vi "Camera controle_PID_CL.vi"() -> ()   [LabVIEW 2026]
uses:
  <vilib>/Serenial/G Industrial Camera/g_industrial_cam/Device Enumeration.ctl
  <vilib>/Serenial/G Industrial Camera/g_industrial_cam/Buffer/Image Size.ctl
  C:/Users/laserfab/Desktop/Cam-PID-LV2026/Thorlabs.MotionControl.Controls.dll
  Thorlabs.MotionControl.Controls.dll
  C:/Users/laserfab/Desktop/Cam-PID-LV2026/Thorlabs.MotionControl.TCube.PiezoCLI.dll
  Thorlabs.MotionControl.TCube.PiezoCLI.dll
  Etat-Data.ctl
  Etat.ctl
  Data-Processing.ctl
  <vilib>/Serenial/G Industrial Camera/g_industrial_cam/Buffer/Buffer.lvclass
  <vilib>/Serenial/G Industrial Camera/g_industrial_cam/Camera/Camera.lvclass
  <vilib>/picture/picture.llb/imagedata.ctl
  Data PID.ctl
  Etat_PID.ctl
  Data Process PID.ctl
  <vilib>/Serenial/G Industrial Camera/g_industrial_cam/Camera/Camera.lvclass/Camera.ctl
  <vilib>/Serenial/G Industrial Camera/g_industrial_cam/Buffer/Buffer.lvclass/Buffer.ctl
  Set CX_CY.ctl
  <vilib>/Serenial/G Industrial Camera/g_industrial_cam/Buffer/Read as Pixmap Mono8.vi
  215a0117-6493-43a3-86db-3e9176a583aa.vi
  <vilib>/Serenial/G Industrial Camera/g_industrial_cam/Camera/GetSetGain.vi
  <vilib>/Serenial/G Industrial Camera/g_industrial_cam/Camera/GetSetExposureTime.vi
  <vilib>/Serenial/G Industrial Camera/g_industrial_cam/Buffer/ReadAsPixmapCore.vi
  <vilib>/Serenial/G Industrial Camera/g_industrial_cam/Camera/Check Not Disconnected.vi
  <vilib>/Utility/error.llb/Error Cluster From Error Code.vi
  <vilib>/Serenial/G Industrial Camera/g_industrial_cam/g_industrial_cam.lvlib
panel:
  out "Refnum de .NET en sortie":refnum<k24>
  out "Acquired Frames/s":dbl=20.37037037037037
  in  "Reset PID 2":bool
  in  "dt (s) PID Axe Y":dbl=0.1 format="%#_13g"
  out "Set CY":dbl=230.26622030324862
  out "CY-offset":dbl=-0.06108959017157645
  in  "Switch Axe Y":bool=TRUE
  in  "PID gains Axe Y":T1={"proportional gain (Kc)"=1.2, "integral time (Ti, min)"=0.01, "derivative time (Td, min)"=0.0}
  in  "Switch Axe X":bool=TRUE
  in  "dt (s) PID Axe X":dbl=0.1 format="%#_13g"
  in  "Activer T-CUbe":bool
  in  "Reset PID":bool
  in  "Activer PID":bool
  out "Set CX":dbl=266.3771356699901
  in  "PID gains Axe X":T1={"proportional gain (Kc)"=0.8, "integral time (Ti, min)"=0.01, "derivative time (Td, min)"=0.0}
  out "CX-offset":dbl=-0.033756492270526905
  in  "Commande onglets":T2(tab)=enum."T-Cube"
  out "Image Caméra":i16[][](graph)
  out "Image ROI":i16[][](graph)
  out "moy Y":dbl=0.005019843768275564 format="%0.4f"
  out "centroid X":dbl(graph)=0.040067485170311556
  out "Centroid Y":dbl(graph)=-0.06325731870961704
  out "sigma X":dbl=0.1236529790065538 caption="écart-type X" format="%0.4f"
  out "moy X":dbl=0.031771673220847445 format="%0.4f"
  out "sigma Y":dbl=0.10913064949168795 caption="écart-type Y" format="%0.4f"
  in  "Pixel size(um)":dbl=5.6
  in  "foc lentille(m)":dbl=1.0
  in  "Switch Pix/urad":bool
  in  "nbre pts sigma":i32=2000
  in  "TCube Axe Y":refnum<k24>(container)
  in  "TCube Axe X":refnum<k24>(container)
  in  "SerialNumber Axe X":string="81843305"
  in  "SerialNumber Axe Y":string="81844014"
  out "Tension Sortie PID Axe Y":dbl(graph)=26.251050201925793
  out "Tension Sortie PID Axe X":dbl(graph)
  in  "Bruit de fond":bool
  out "Sensor Size":T3={"Width"=659, "Height"=494}
  in  "Set Centroid":bool
  in  "Shutter (us)":dbl(knob)=1000.0 scale=22.0..10000000.0
  in  "Save Image":bool
  in  "Gain Caméra":i32(knob)=2 scale=0.0..1023.0
  in  "Start /Stop Acquisition":bool
  out "Etat":string="Programme Arrêté"
  out "Devices":T4[](array[typedef])=[{"ID"="Basler-acA640-121gm-40025274", "Protocol"="GigEVision", "Vendor"="Basler", "Model"="acA640-121gm", "Serial"="40025274", "Address"="192.168.3.4"}, {"ID"="Basler-acA640-121gm-40135516", "Protocol"="GigEVision", "Vendor"="Basler", "Model"="acA640-121gm", "Serial"="40135516", "Address"="192.168.3.3"}]
  in  "stop":bool
  out "error out":errorcluster
  # "Commande PID"
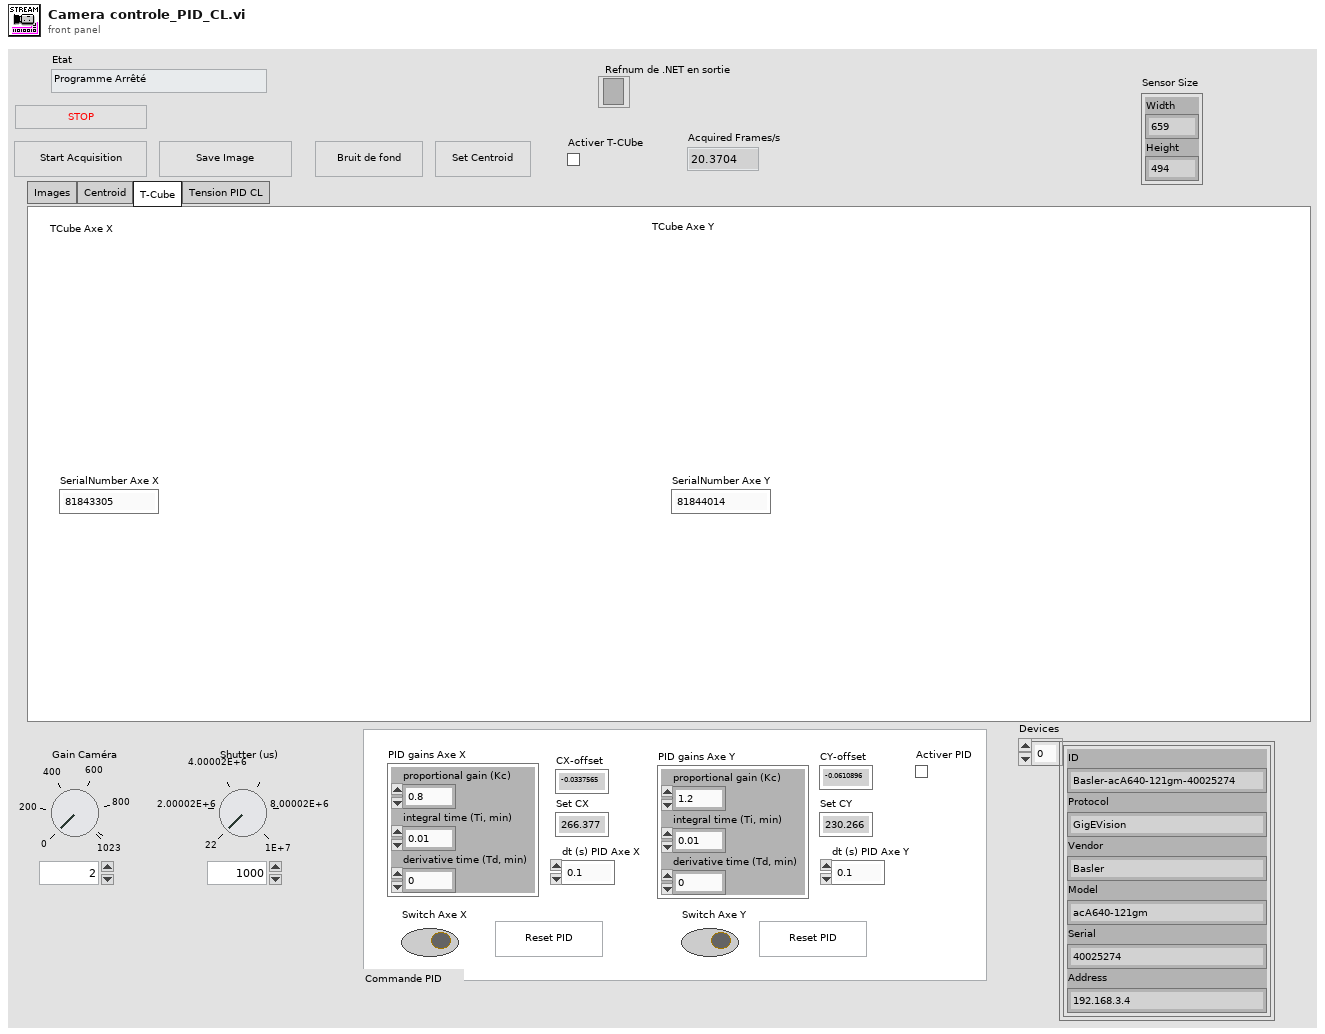
[diagram p1: front panel]
types:
  T1 = cluster{"proportional gain (Kc)":dbl, "integral time (Ti, min)":dbl, "derivative time (Td, min)":dbl}
  T2 = enum32{"Images", "Centroid", "T-Cube", "Tension PID CL"}
  T3 = typedef "g_industrial_cam.lvlib/Buffer.lvclass/Image Size.ctl" = cluster{"Width":u16, "Height":u16}
  T4 = typedef "g_industrial_cam.lvlib/Device Enumeration.ctl" = cluster{"ID":string, "Protocol":string, "Vendor":string, "Model":string, "Serial":string, "Address":string}
  T5 = typedef "Data Process PID.ctl" = cluster{"Pos Init CX":dbl, "Pos Init CY":dbl}
  T6 = typedef "Data PID.ctl" = cluster{"Etat PID":T7, "Data PID":variant}
  T7 = typedef "Etat_PID.ctl" = enum16{"PID", "Stop", "Reset PID", "Set Centroid", "Set T-Cube"}
  T8 = typedef "Data-Processing.ctl" = cluster{"Acqu?":bool, "Image Caméra":picture, "Image Data":T9, "Image brut":i16[][], "BKG":i16[][], "Image -BKG":i16[][], "Offset Centroid X":dbl, "Offset Centroid Y":dbl, "Centroid X-offset":dbl, "Centroid Y-offset":dbl, "Refnum GraphInt":refnum<vi>, "Refnum ROI":refnum<vi>, "Buffer en sortie":refnum<class "Buffer.lvclass">, "Camera":refnum<class "Camera.lvclass">, "Centroid X current":dbl, "Centroid Y current":dbl, "Gain Caméra":i32, "Shutter (us)":dbl, "Refnum Gain":refnum<vi>, "Refnum Shutter":refnum<vi>, "sigma Y":dbl, "mean Y":dbl, "mean X":dbl, "sigma X":dbl, "Référence T-Cube":T10}
  T9 = typedef "imagedata.ctl" = cluster{"image type":i32, "image depth":i32, "image":u8[], "mask":u8[], "colors":u32[], "Rectangle":cluster{"left":i16, "top":i16, "right":i16, "bottom":i16}}
  T10 = typedef "Référence T-Cube.ctl" = cluster{"T-Cube X":refnum<k24>, "T-Cube Y":refnum<k24>}
  T11 = typedef "Etat.ctl" = enum16{"Initialiser", "Start Acquisition", "Stop Acquisition", "Stop Prog", "Shutter", "Gain", "BKG", "Set Centroid", "Activer T-Cube", "Save Image"}
  T12 = typedef "Etat-Data.ctl" = cluster{"Etat":T11, "Data":variant}
  T13 = typedef "Set CX_CY.ctl" = cluster{"CX":dbl, "CY":dbl}
  T14 = cluster{"C0PX":dbl, "C0PY":dbl, "C1PX":dbl, "C1PY":dbl}
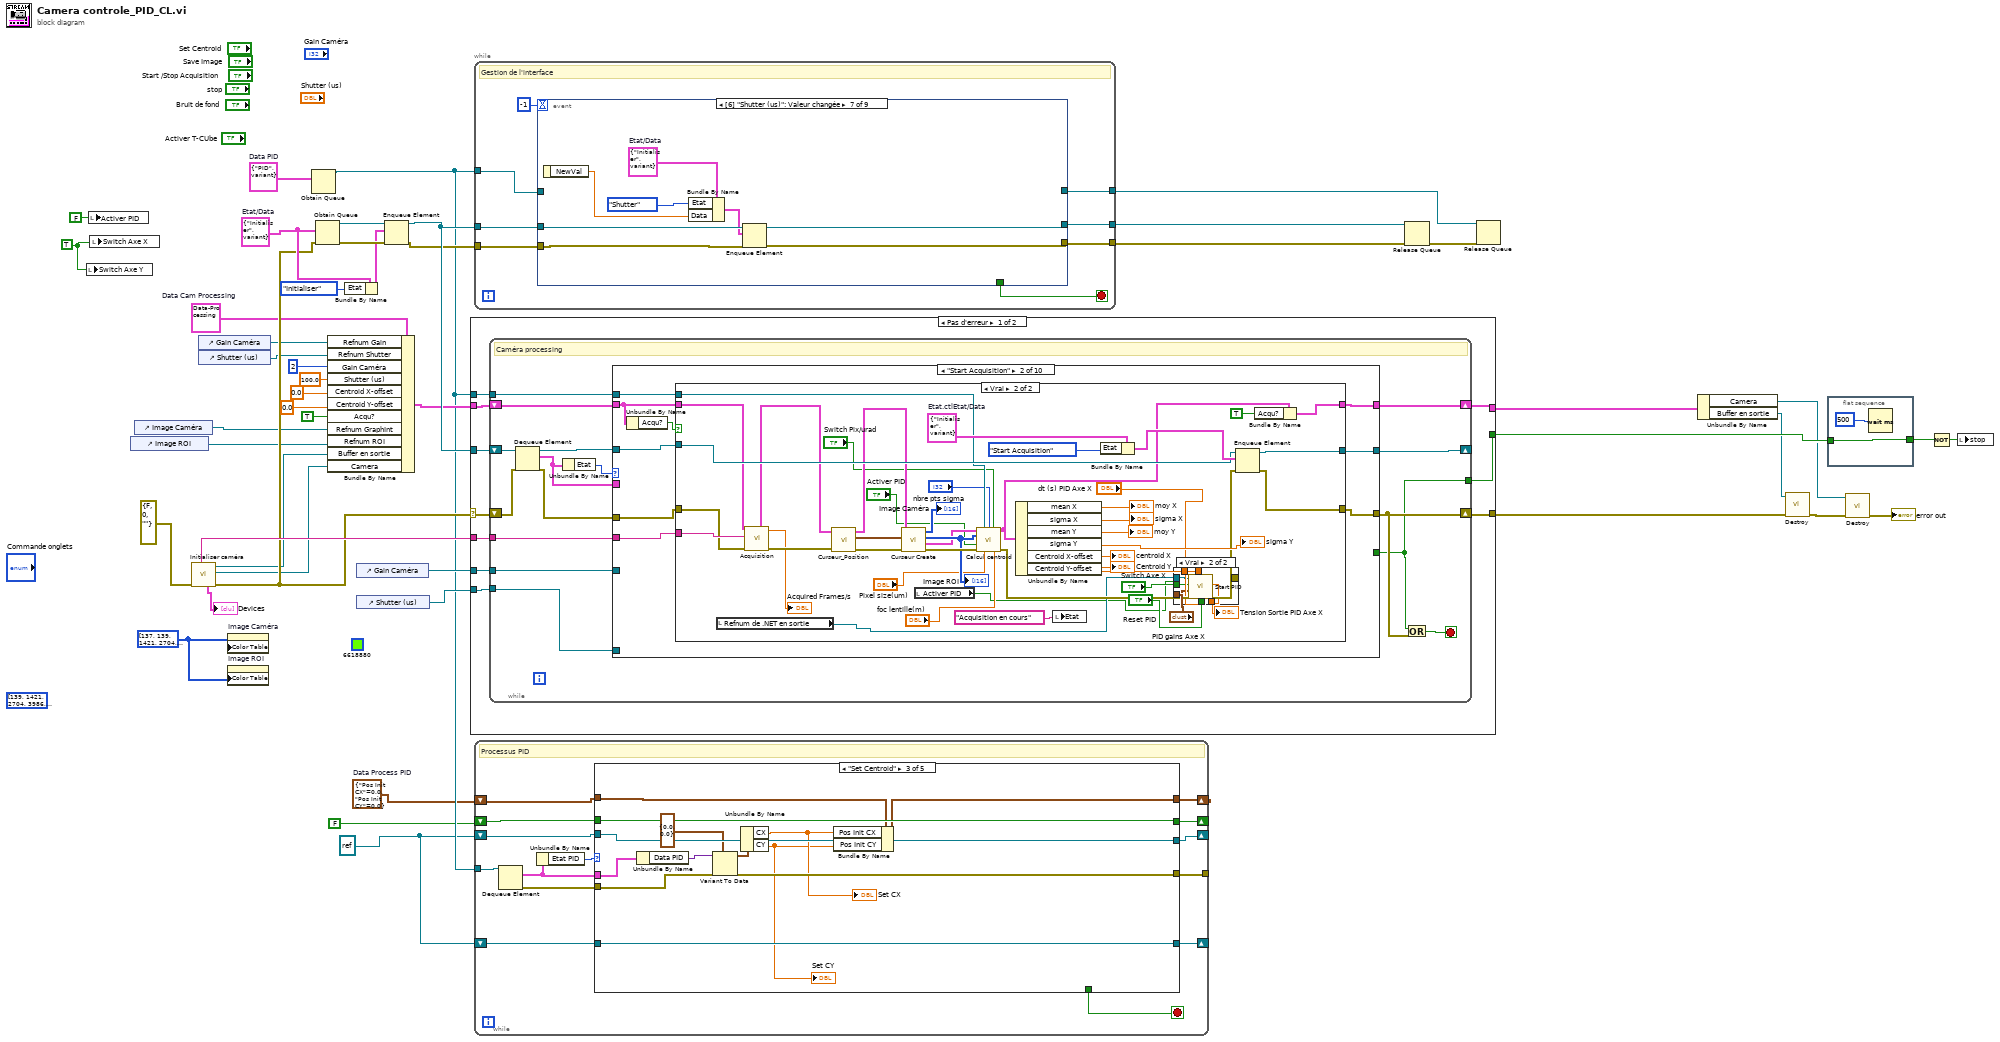
[diagram p0: block diagram]
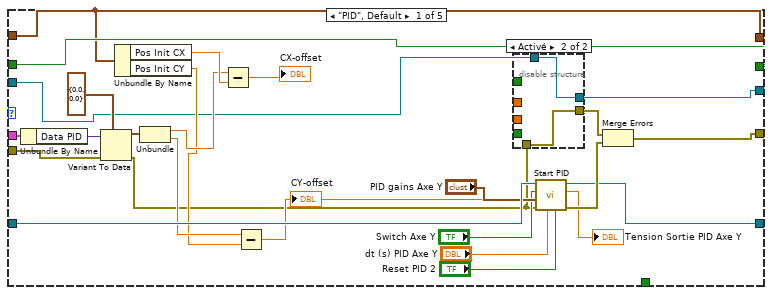
[diagram p2: hidden frame]
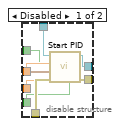
[diagram p3: hidden frame]
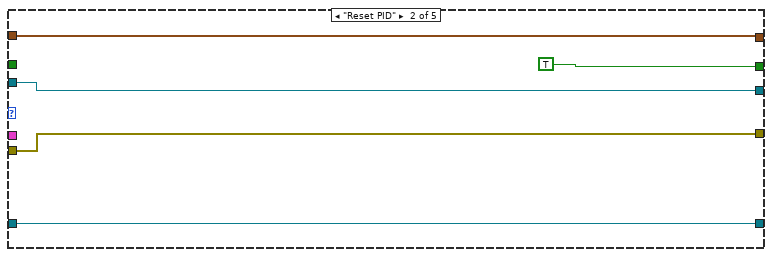
[diagram p4: hidden frame]
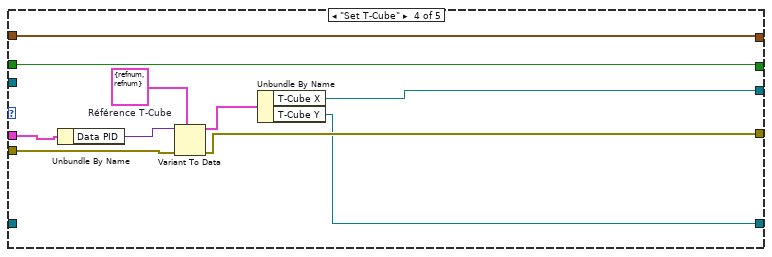
[diagram p5: hidden frame]
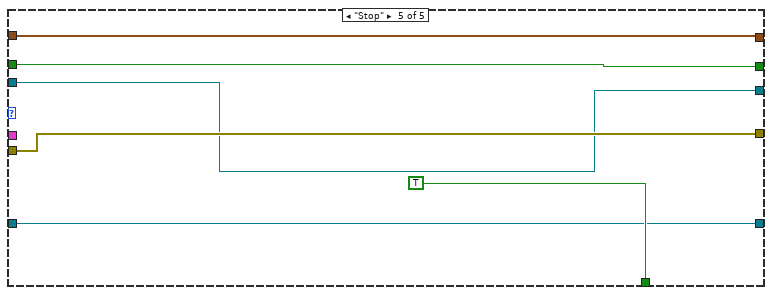
[diagram p6: hidden frame]
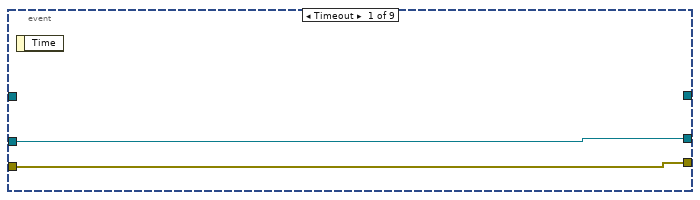
[diagram p7: hidden frame]
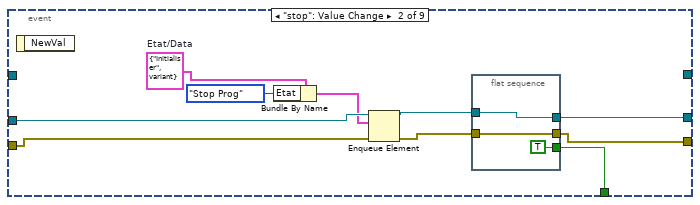
[diagram p8: hidden frame]
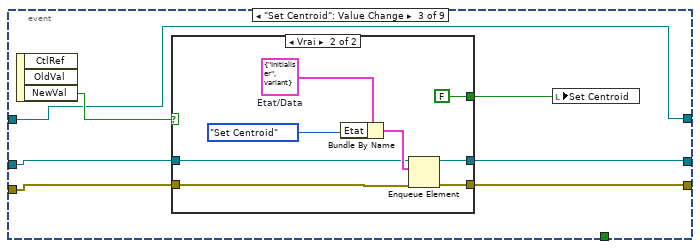
[diagram p9: hidden frame]
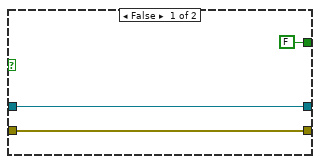
[diagram p10: hidden frame]
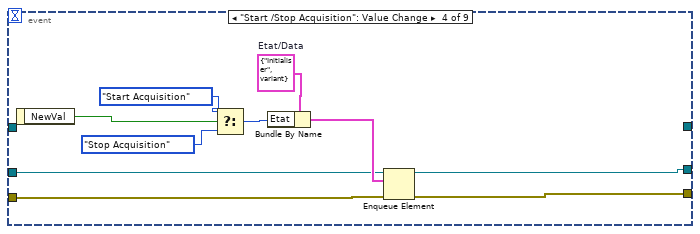
[diagram p11: hidden frame]
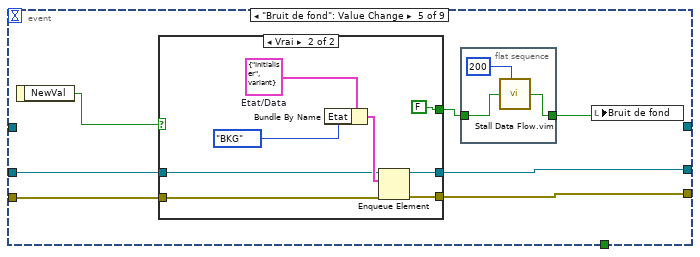
[diagram p12: hidden frame]
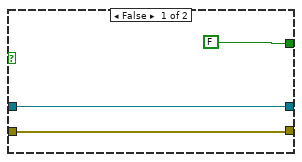
[diagram p13: hidden frame]
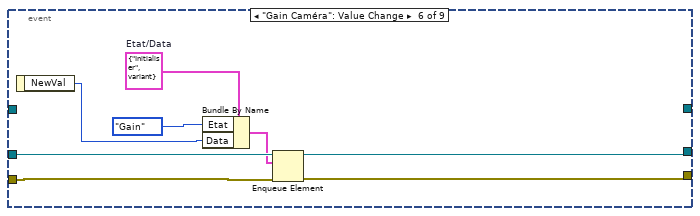
[diagram p14: hidden frame]
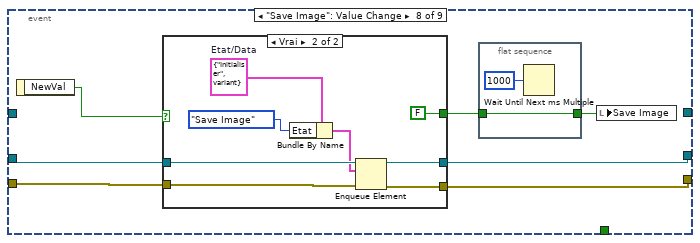
[diagram p15: hidden frame]
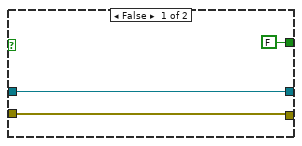
[diagram p16: hidden frame]
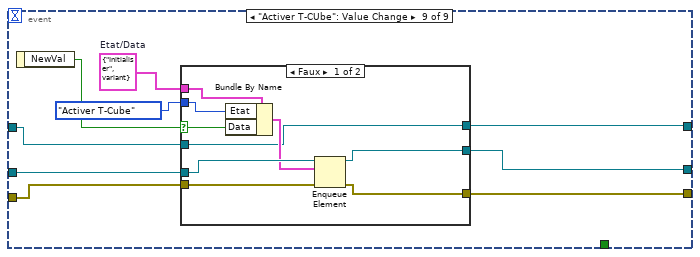
[diagram p17: hidden frame]
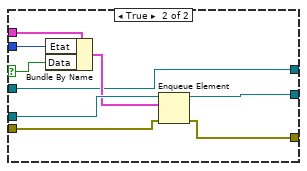
[diagram p18: hidden frame]
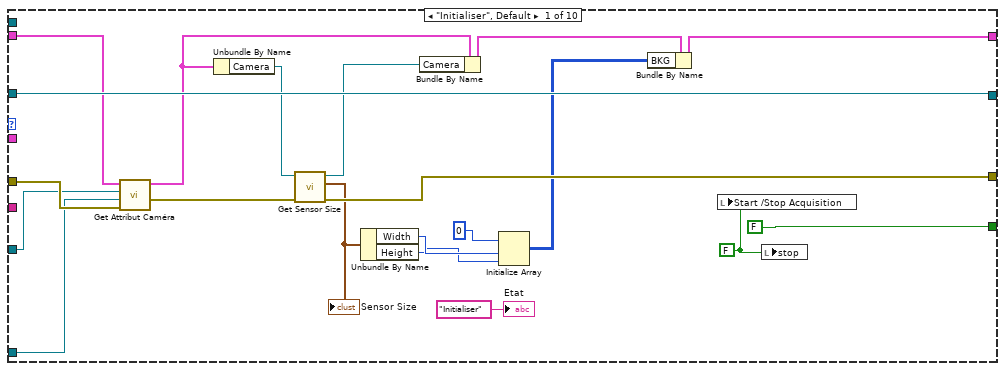
[diagram p19: hidden frame]
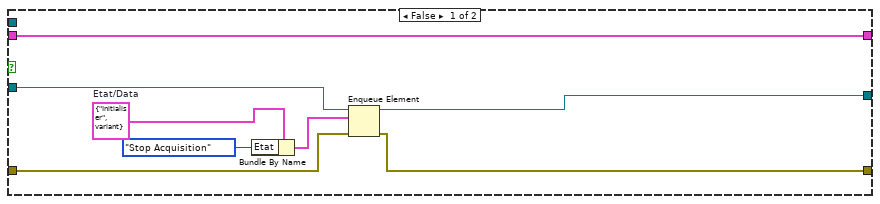
[diagram p20: hidden frame]
diagram:
  w5 = TRUE ("Activer PID")
  w6 = refnum<k24> refnum ("Device")
  w8 = T5 {"Pos Init CX"=0.0, "Pos Init CY"=0.0}  # Data Process PID
  w13 = T6 {"Etat PID"=enum."PID", "Data PID"=variant}  # Data PID
  w20 = u32[] [137, 139, 1421, 2704, 3986, 5268, 6550, 7833, 9115, 10397, 11679, 12962, 14244, 15526, 16809, 18091, 19373, 20655, 21938, 23220, 24502, 25784, 27067, 28349, 29631, 30914, 32196, 33478, 34760, 36043, 37325, 38607, 39890, 41172, 42454, 43736, 45019, 46301, 47583, 48865, 50148, 51430, 52712, 53995, 55277, 56559, 57841, 59124, 60406, 61688, 62970, 64253, 65535, 65530, 65525, 65520, 65515, 65510, 65505, 65500, 65495, 65490, 65485, 65480, 65475, 65470, 65465, 65460, 65455, 65450, 65445, 65440, 65435, 65430, 65425, 65420, 65415, 65410, 65405, 65400, 65395, 65390, 65385, 65380, 65375, 65370, 65365, 65360, 65355, 65350, 65345, 65340, 65335, 65330, 65325, 65320, 65315, 65310, 65305, 65300, 65295, 65290, 65285, 65280, 392960, 720640, 1048320, 1376000, 1703680, 2031360, 2359040, 2686720, 3014400, 3342080, 3669760, 3997440, 4325120, 4652800, 4980480, 5308160, 5635840, 5963520, 6291200, 6618880, 6946560, 7274240, 7601920, 7929600, 8257280, 8584960, 8912640, 9240320, 9568000, 9895680, 10223360, 10551040, 10878720, 11206400, 11534080, 11861760, 12189440, 12517120, 12844800, 13172480, 13500160, 13827840, 14155520, 14483200, 14810880, 15138560, 15466240, 15793920, 16121600, 16449280, 16776960, 16775680, 16774400, 16773120, 16771840, 16770560, 16769280, 16768000, 16766720, 16765440, 16764160, 16762880, 16761600, 16760320, 16759040, 16757760, 16756480, 16755200, 16753920, 16752640, 16751360, 16750080, 16748800, 16747520, 16746240, 16744960, 16743680, 16742400, 16741120, 16739840, 16738560, 16737280, 16736000, 16734720, 16733440, 16732160, 16730880, 16729600, 16728320, 16727040, 16725760, 16724480, 16723200, 16721920, 16720640, 16719360, 16718080, 16716800, 16715520, 16714240, 16712960, 16711680, 16712965, 16714250, 16715535, 16716820, 16718105, 16719390, 16720675, 16721960, 16723245, 16724530, 16725815, 16727100, 16728385, 16729670, 16730955, 16732240, 16733525, 16734810, 16736095, 16737380, 16738665, 16739950, 16741235, 16742520, 16743805, 16745090, 16746375, 16747660, 16748945, 16750230, 16751515, 16752800, 16754085, 16755370, 16756655, 16757940, 16759225, 16760510, 16761795, 16763080, 16764365, 16765650, 16766935, 16768220, 16769505, 16770790, 16772075, 16773360, 16774645, 16775930, 16777215] ("Tableau 3")
  (unwired) u32[] [139, 1421, 2704, 3986, 5268, 6550, 7833, 9115, 10397, 11679, 12962, 14244, 15526, 16809, 18091, 19373, 20655, 21938, 23220, 24502, 25784, 27067, 28349, 29631, 30914, 32196, 33478, 34760, 36043, 37325, 38607, 39890, 41172, 42454, 43736, 45019, 46301, 47583, 48865, 50148, 51430, 52712, 53995, 55277, 56559, 57841, 59124, 60406, 61688, 62970, 64253, 65535, 65530, 65525, 65520, 65515, 65510, 65505, 65500, 65495, 65490, 65485, 65480, 65475, 65470, 65465, 65460, 65455, 65450, 65445, 65440, 65435, 65430, 65425, 65420, 65415, 65410, 65405, 65400, 65395, 65390, 65385, 65380, 65375, 65370, 65365, 65360, 65355, 65350, 65345, 65340, 65335, 65330, 65325, 65320, 65315, 65310, 65305, 65300, 65295, 65290, 65285, 65280, 392960, 720640, 1048320, 1376000, 1703680, 2031360, 2359040, 2686720, 3014400, 3342080, 3669760, 3997440, 4325120, 4652800, 4980480, 5308160, 5635840, 5963520, 6291200, 6618880, 6946560, 7274240, 7601920, 7929600, 8257280, 8584960, 8912640, 9240320, 9568000, 9895680, 10223360, 10551040, 10878720, 11206400, 11534080, 11861760, 12189440, 12517120, 12844800, 13172480, 13500160, 13827840, 14155520, 14483200, 14810880, 15138560, 15466240, 15793920, 16121600, 16449280, 16776960, 16775680, 16774400, 16773120, 16771840, 16770560, 16769280, 16768000, 16766720, 16765440, 16764160, 16762880, 16761600, 16760320, 16759040, 16757760, 16756480, 16755200, 16753920, 16752640, 16751360, 16750080, 16748800, 16747520, 16746240, 16744960, 16743680, 16742400, 16741120, 16739840, 16738560, 16737280, 16736000, 16734720, 16733440, 16732160, 16730880, 16729600, 16728320, 16727040, 16725760, 16724480, 16723200, 16721920, 16720640, 16719360, 16718080, 16716800, 16715520, 16714240, 16712960, 16711680, 16712965, 16714250, 16715535, 16716820, 16718105, 16719390, 16720675, 16721960, 16723245, 16724530, 16725815, 16727100, 16728385, 16729670, 16730955, 16732240, 16733525, 16734810, 16736095, 16737380, 16738665, 16739950, 16741235, 16742520, 16743805, 16745090, 16746375, 16747660, 16748945, 16750230, 16751515, 16752800, 16754085, 16755370, 16756655, 16757940, 16759225, 16760510, 16761795, 16763080, 16764365, 16765650, 16766935, 16768220, 16769505, 16770790, 16772075, 16773360, 16774645, 16775930, 16777215] ("Tableau")
  (unwired) u32 6618880 ("color(black)")
  w28 = T8 {"Acqu?"=FALSE, "Image Caméra"=bytes[0], "Image Data"={"image type"=0, "image depth"=0, "image"=[], "mask"=[], "colors"=[], "Rectangle"={"left"=0, "top"=0, "right"=0, "bottom"=0}}, "Image brut"=[], "BKG"=[], "Image -BKG"=[], "Offset Centroid X"=0.0, "Offset Centroid Y"=0.0, "Centroid X-offset"=0.0, "Centroid Y-offset"=0.0, "Refnum GraphInt"=refnum, "Refnum ROI"=refnum, "Buffer en sortie"=refnum, "Camera"=refnum, "Centroid X current"=0.0, "Centroid Y current"=0.0, "Gain Caméra"=0, "Shutter (us)"=0.0, "Refnum Gain"=refnum, "Refnum Shutter"=refnum, "sigma Y"=0.0, "mean Y"=0.0, "mean X"=0.0, "sigma X"=0.0, "Référence T-Cube"={"T-Cube X"=refnum, "T-Cube Y"=refnum}}  # Data Cam Processing
  w40 = T12 {"Etat"=enum."Initialiser", "Data"=variant}  # Etat/Data
  n1 = local write "Switch Axe Y"(w5) -> ()
  n2 = local write "Activer PID"(FALSE ("Activer PID")) -> ()
  n3 = local write "Switch Axe X"(w5) -> ()
  n4 = control-ref of="Image ROI"() -> (w19:refnum<vi>)
  n5 = control-ref of="Image Caméra"() -> (w23:refnum<vi>)
  n6 = call "Initialiser caméra.vi"("entrée d'erreur (pas d'erreur)"=errorcluster {"status"=FALSE, "code"=0, "source"=""}) -> ("sortie d'erreur"=w29:errorcluster, "Camera"=w17:refnum<class "Camera.lvclass">, "Buffer en sortie"=w18:refnum<class "Buffer.lvclass">, "Devices"=→"Devices":T4[], "Pixel Format"=w46:string)  [unwired: 5 in, 1 out]
  n7 = control-ref of="Gain Caméra"() -> (w2:refnum<vi>)
  n8 = control-ref of="Shutter (us)"() -> (w1:refnum<vi>)
  n9 = property on="Image Caméra" class="GraphInt (strict)"("Color Table"=w20) -> ()  [unwired: 2 in, 2 out]
  n10 = property on="Image ROI" class="GraphInt (strict)"("Color Table"=w20) -> ()  [unwired: 2 in, 2 out]
  n11 = Obtain Queue(element data type=w13) -> (queue out=w10:refnum<queue>)  [unwired: 4 in, 2 out]
  n12 = Obtain Queue(element data type=w40, error in (no error)=w29) -> (queue out=w41:refnum<queue>, error out=w42:errorcluster)  [unwired: 3 in, 1 out]
  n13 = Bundle By Name(cluster=w28, "Refnum Gain"=w2, "Refnum Shutter"=w1, "Gain Caméra"=2, "Shutter (us)"=100.0, "Centroid X-offset"=0.0 ("Centroid X"), "Centroid Y-offset"=0.0 ("Centroid Y"), "Acqu?"=TRUE, "Refnum GraphInt"=w23, "Refnum ROI"=w19, "Buffer en sortie"=w18, "Camera"=w17) -> (w27:T8)
  n14 = Bundle By Name(cluster=w40, "Etat"=Etat."Initialiser") -> (w39:T12)
  n15 = control-ref of="Gain Caméra"() -> (w25:refnum<vi>)
  n16 = control-ref of="Shutter (us)"() -> (w24:refnum<vi>)
  n17 = Enqueue Element(queue=w41, element=w39, error in (no error)=w42) -> (queue out=w37:refnum<queue>, error out=w35:errorcluster)  [unwired: 1 in, 1 out]
  n18 = case shown="Pas d'erreur" w29 {
    selector: w29 -> [w57 w293]
    tunnel: [w56 w293] -> w45
    tunnel: w46 -> [w55 _]
    tunnel: w37 -> [w54 _]
    tunnel: [w53 FALSE ("stop")] -> w32
    tunnel: w27 -> [w52 w291]
    tunnel: w25 -> [w51 _]
    tunnel: w24 -> [w50 _]
    tunnel: [w49 w291] -> w16
    tunnel: w10 -> [w48 _]
    frame No Error {
      n19 = while {
        shift-right: [w72] -> w56
        shift-left: w57 -> [w69]
        tunnel: w55 -> [w71]
        shift-right: [w65] -> _
        shift-left: w54 -> [w70]
        tunnel: [w64] -> w53
        shift-right: [w62] -> w49
        shift-left: w52 -> [w61]
        tunnel: w51 -> [w60]
        tunnel: w50 -> [w59]
        tunnel: w48 -> [w58]
        stop <- w73 stop-if-true
        # "Caméra processing"
        n20 = Dequeue Element(queue=w70, error in (no error)=w69) -> (queue out=w66:refnum<queue>, element=w63:T12, error out=w68:errorcluster)  [unwired: 1 in, 1 out]
        n21 = Unbundle By Name(w63) -> ("Etat"=w67:T11)
        n22 = case shown="\"Start Acquisition\"" w67 {
          tunnel: [w85 w102 w170 w186 w197 w211 w226 w236 w241 w264] -> w72
          tunnel: w71 -> [_ w101 _ _ _ _ _ _ _ _]
          tunnel: w68 -> [w90 w100 w169 w187 w203 w216 w225 w236 w242 w262]
          tunnel: w66 -> [w93 w98 w171 w192 w205 w218 w231 w235 w249 w266]
          tunnel: [w93 w99 w172 w192 w205 w218 w231 w235 w249 w266] -> w65
          tunnel: [FALSE _ FALSE ("stop") TRUE ("stop") _ _ _ _ _ _] -> w64
          tunnel: w63 -> [_ _ _ _ w204 w217 _ _ _ w263]
          tunnel: [w84 w95 w166 w189 w194 w209 w220 w233 w248 w251] -> w62
          tunnel: w61 -> [w76 w96 w167 w189 w196 w208 w222 w234 w247 w250]
          tunnel: w60 -> [w88 _ _ _ _ _ _ _ _ _]
          tunnel: w59 -> [w87 _ _ _ _ _ _ _ _ _]
          tunnel: w58 -> [_ w94 _ w188 _ _ _ _ w246 w255]
          frame "Initialiser", Default {
            w89 = FALSE ("stop")
            n23 = call "Get Attribut Caméra.vi"("entrée d'erreur (pas d'erreur)"=w90, "Shutter Caméra"=w87, "Gain Caméra"=w88, "Data Cam Processing"=w76) -> ("sortie d'erreur"=w86:errorcluster, "Data Cam Processing out"=w75:T8)  [unwired: 6 in]
            n24 = Unbundle By Name(w75) -> ("Camera"=w74:refnum<class "Camera.lvclass">)
            n25 = call <vilib>:"Get Sensor Size.vi"("error in (no error)"=w86, "Camera in"=w74) -> ("error out"=w85:errorcluster, "Sensor Size"=w83:T3, "Camera"=w77:refnum<class "Camera.lvclass">)  [unwired: 7 in]
            "Sensor Size" <- w83
            n26 = Unbundle By Name(w83) -> ("Width"=w81:u16, "Height"=w80:u16)
            n27 = Bundle By Name(cluster=w75, "Camera"=w77) -> (w78:T8)
            n28 = Initialize Array(u8 0, w81, w80) -> (w79:u8[][])
            n29 = Bundle By Name(cluster=w78, "BKG"=w79) -> (w84:T8)
            n30 = local write "Start /Stop Acquisition"(w89) -> ()
            n31 = local write "stop"(w89) -> ()
            "Etat" <- "Initialiser" ("Etat")
          }
          frame "Start Acquisition" {
            n32 = Unbundle By Name(w96) -> ("Acqu?"=w97:bool)
            n33 = case shown="Vrai" w97 {
              tunnel: [w107 w152] -> w102
              tunnel: w101 -> [_ w154]
              tunnel: w100 -> [w108 w153]
              tunnel: [w109 w148] -> w99
              tunnel: w98 -> [w110 w149]
              tunnel: w96 -> [w103 w143]
              tunnel: [w103 w146] -> w95
              tunnel: w94 -> [_ w131]
              frame False {
                w106 = T12 {"Etat"=enum."Initialiser", "Data"=variant}  # Etat/Data
                n34 = Bundle By Name(cluster=w106, "Etat"=Etat."Stop Acquisition") -> (w105:T12)
                n35 = Enqueue Element(queue=w110, element=w105, error in (no error)=w108) -> (queue out=w109:refnum<queue>, error out=w107:errorcluster)  [unwired: 1 in, 1 out]
              }
              frame True {
                w151 = T12 {"Etat"=enum."Initialiser", "Data"=variant}  # Etat.ctlEtat/Data
                n36 = local read "Refnum de .NET en sortie"() -> (w112:refnum<k24>)
                n37 = call "Acquisition.vi"("Data Cam Processing en entrée"=w143, "entrée d'erreur"=w153, "Pixel Format"=w154) -> ("sortie d'erreur"=w142:errorcluster, "Acquired Frames/s"=→"Acquired Frames/s":dbl, "Data Cam Processing en sortie"=w135:T8)  [unwired: 5 in, 1 out]
                n38 = call "Curseur_Position.vi"("error in (no error)"=w142, "Data Cam Processing"=w135) -> ("error out"=w140:errorcluster, "Curseur"=w141:T14, "Data Cam Processing 2"=w136:T8)  [unwired: 7 in]
                n39 = call "Curseur Create.vi"("error in (no error)"=w140, "Data Cam Processing"=w136, "Curseur"=w141) -> ("error out"=w139:errorcluster, "Data Cam Processing out"=w134:T8, "Img ROI"=w137:i16[][], "Image Out"=→"Image Caméra":i16[][])  [unwired: 5 in]
                "Image ROI" <- w137
                n40 = local read "Activer PID"() -> (w111:bool)
                n41 = call "Calcul centroid.vi"("Data Cam Processing"=w134, "Data PID"=w131, "sample length"="nbre pts sigma", "Switch Pix/um"="Switch Pix/urad", "ROI"=w137, "Activer PID"="Activer PID", "error in (no error)"=w139, "Pixel size(um)"="Pixel size(um)", "foc lentille"="foc lentille(m)") -> ("Data Cam Processing 2"=w133:T8, "error out"=w120:errorcluster)  [unwired: 3 in, 2 out]
                n42 = Unbundle By Name(w133) -> ("mean X"=→"moy X":dbl, "sigma X"=→"sigma X":dbl, "mean Y"=→"moy Y":dbl, "sigma Y"=→"sigma Y":dbl, "Centroid X-offset"=w116:dbl, "Centroid Y-offset"=→"Centroid Y":dbl)
                "centroid X" <- w116
                n43 = local write "Etat"("Acquisition en cours" ("Etat")) -> ()
                n44 = Bundle By Name(cluster=w151, "Etat"=Etat."Start Acquisition") -> (w150:T12)
                n45 = case shown="Vrai" w111 {
                  tunnel: w120 -> [w155 w164]
                  tunnel: [w155 w163] -> w119
                  tunnel: "dt (s) PID Axe X" -> [_ w162]
                  tunnel: "PID gains Axe X" -> [_ w161]
                  tunnel: w116 -> [_ w160]
                  tunnel: "Switch Axe X" -> [_ w159]
                  tunnel: [_ w158] -> w114
                  tunnel: "Reset PID" -> [_ w157]
                  tunnel: w112 -> [_ w156]
                  frame False {
                  }
                  frame True {
                    n46 = call "Start PID.vi"("Reset PID en entrée"=w157, "dt (s) PID"=w162, "Centroid Variable"=w160, "entrée d'erreur (pas d'erreur)"=w164, "PID gains"=w161, "Switch Axe"=w159, "Refnum de .NET en entrée"=w156) -> ("sortie d'erreur"=w163:errorcluster, "Tension Sortie PID"=w158:dbl)  [unwired: 2 in, 1 out]
                  }
                }
                "Tension Sortie PID Axe X" <- w114
                n47 = Enqueue Element(queue=w149, element=w150, error in (no error)=w119) -> (queue out=w148:refnum<queue>, error out=w152:errorcluster)  [unwired: 1 in, 1 out]
                n48 = Bundle By Name(cluster=w133, "Acqu?"=TRUE) -> (w146:T8)
              }
            }
          }
          frame "Stop Acquisition" {
            n49 = Unbundle By Name(w167) -> ("Acqu?"=w168:bool)
            n50 = case shown="Vrai" w168 {
              tunnel: [w177 w182] -> w172
              tunnel: w171 -> [w177 w182]
              tunnel: [w176 w181] -> w170
              tunnel: w169 -> [w176 w181]
              tunnel: w167 -> [w174 w180]
              tunnel: [w173 w179] -> w166
              frame False {
                n51 = Bundle By Name(cluster=w174, "Acqu?"=TRUE) -> (w173:T8)
              }
              frame True {
                n52 = Bundle By Name(cluster=w180, "Acqu?"=FALSE) -> (w179:T8)
              }
            }
          }
          frame "Stop Prog" {
            w185 = T6 {"Etat PID"=enum."PID", "Data PID"=variant}  # Data PID
            n53 = local write "Etat"("Programme Arrêté" ("Etat")) -> ()
            n54 = Bundle By Name(cluster=w185, "Etat PID"=Etat_PID."Stop") -> (w184:T6)
            n55 = Enqueue Element(queue=w188, element=w184, error in (no error)=w187) -> (error out=w186:errorcluster)  [unwired: 1 in, 2 out]
          }
          frame "Gain" {
            n56 = Unbundle By Name(w204) -> ("Data"=w202:variant)
            n57 = local write "Etat"("Gain" ("Etat")) -> ()
            n58 = Unbundle By Name(w196) -> ("Camera"=w195:refnum<class "Camera.lvclass">)
            n59 = Variant To Data(error in=w203, type=0, Variant=w202) -> (data=w199:i32, error out=w198:errorcluster)
            n60 = call <vilib>:"Set Gain.vi"("error in (no error)"=w198, "Gain"=w199, "Camera in"=w195) -> ("error out"=w197:errorcluster, "Camera"=w193:refnum<class "Camera.lvclass">)  [unwired: 7 in]
            n61 = Bundle By Name(cluster=w196, "Camera"=w193) -> (w194:T8)
          }
          frame "Shutter" {
            n62 = Unbundle By Name(w217) -> ("Data"=w215:variant)
            n63 = local write "Etat"("Shutter" ("Etat")) -> ()
            n64 = Variant To Data(error in=w216, type=0.0, Variant=w215) -> (data=w210:dbl, error out=w212:errorcluster)
            n65 = Unbundle By Name(w208) -> ("Camera"=w207:refnum<class "Camera.lvclass">)
            n66 = call <vilib>:"Set Exposure Time.vi"("error in (no error)"=w212, "Time (us)"=w210, "Camera in"=w207) -> ("error out"=w211:errorcluster, "Camera"=w206:refnum<class "Camera.lvclass">)  [unwired: 7 in]
            n67 = Bundle By Name(cluster=w208, "Camera"=w206) -> (w209:T8)
          }
          frame "Save Image" {
            n68 = Unbundle By Name(w222) -> ("Buffer en sortie"=w221:refnum<class "Buffer.lvclass">)
            n69 = call-poly <vilib>:"Read as Pixmap.vi"("Colours (Empty: Use Greyscale)"=u32[] [139, 1421, 2704, 3986, 5268, 6550, 7833, 9115, 10397, 11679, 12962, 14244, 15526, 16809, 18091, 19373, 20655, 21938, 23220, 24502, 25784, 27067, 28349, 29631, 30914, 32196, 33478, 34760, 36043, 37325, 38607, 39890, 41172, 42454, 43736, 45019, 46301, 47583, 48865, 50148, 51430, 52712, 53995, 55277, 56559, 57841, 59124, 60406, 61688, 62970, 64253, 65535, 65530, 65525, 65520, 65515, 65510, 65505, 65500, 65495, 65490, 65485, 65480, 65475, 65470, 65465, 65460, 65455, 65450, 65445, 65440, 65435, 65430, 65425, 65420, 65415, 65410, 65405, 65400, 65395, 65390, 65385, 65380, 65375, 65370, 65365, 65360, 65355, 65350, 65345, 65340, 65335, 65330, 65325, 65320, 65315, 65310, 65305, 65300, 65295, 65290, 65285, 65280, 392960, 720640, 1048320, 1376000, 1703680, 2031360, 2359040, 2686720, 3014400, 3342080, 3669760, 3997440, 4325120, 4652800, 4980480, 5308160, 5635840, 5963520, 6291200, 6618880, 6946560, 7274240, 7601920, 7929600, 8257280, 8584960, 8912640, 9240320, 9568000, 9895680, 10223360, 10551040, 10878720, 11206400, 11534080, 11861760, 12189440, 12517120, 12844800, 13172480, 13500160, 13827840, 14155520, 14483200, 14810880, 15138560, 15466240, 15793920, 16121600, 16449280, 16776960, 16775680, 16774400, 16773120, 16771840, 16770560, 16769280, 16768000, 16766720, 16765440, 16764160, 16762880, 16761600, 16760320, 16759040, 16757760, 16756480, 16755200, 16753920, 16752640, 16751360, 16750080, 16748800, 16747520, 16746240, 16744960, 16743680, 16742400, 16741120, 16739840, 16738560, 16737280, 16736000, 16734720, 16733440, 16732160, 16730880, 16729600, 16728320, 16727040, 16725760, 16724480, 16723200, 16721920, 16720640, 16719360, 16718080, 16716800, 16715520, 16714240, 16712960, 16711680, 16712965, 16714250, 16715535, 16716820, 16718105, 16719390, 16720675, 16721960, 16723245, 16724530, 16725815, 16727100, 16728385, 16729670, 16730955, 16732240, 16733525, 16734810, 16736095, 16737380, 16738665, 16739950, 16741235, 16742520, 16743805, 16745090, 16746375, 16747660, 16748945, 16750230, 16751515, 16752800, 16754085, 16755370, 16756655, 16757940, 16759225, 16760510, 16761795, 16763080, 16764365, 16765650, 16766935, 16768220, 16769505, 16770790, 16772075, 16773360, 16774645, 16775930, 16777215] ("Tableau"), "error in (no error)"=w225, "Buffer in"=w221) -> ("Image Data"=w223:T9, "Buffer"=w219:refnum<class "Buffer.lvclass">)  [unwired: 6 in, 1 out]
            n70 = call <vilib>:"Application Directory.vi"() -> ("Application Directory"=w229:path)
            n71 = Build Path(base path=w229, name or relative path=path "img.png" ("nom ou chemin relatif")) -> (appended path=w227:path)
            n72 = call <vilib>:"Write PNG File.vi"("image data"=w223, "path to PNG file"=w227) -> ("error out"=w226:errorcluster)  [unwired: 8 in, 1 out]
            n73 = Bundle By Name(cluster=w222, "Buffer en sortie"=w219) -> (w220:T8)
            n74 = local write "Etat"("Image enregistrée" ("Etat")) -> ()
          }
          frame "BKG" {
            n75 = Unbundle By Name(w234) -> ("Image brut"=w232:i16[][])
            n76 = Bundle By Name(cluster=w234, "BKG"=w232) -> (w233:T8)
          }
          frame "Set Centroid" {
            w245 = T6 {"Etat PID"=enum."PID", "Data PID"=variant}  # Data PID
            n77 = Unbundle By Name(w247) -> ("Centroid X current"=w238:dbl, "Centroid Y current"=w237:dbl)
            n78 = Bundle By Name(cluster=T13 {"CX"=0.0, "CY"=0.0}, "CX"=w238, "CY"=w237) -> (w239:T13)
            n79 = Bundle By Name(cluster=w247, "Offset Centroid X"=w238, "Offset Centroid Y"=w237) -> (w248:T8)
            n80 = Bundle By Name(cluster=w245, "Etat PID"=Etat_PID."Set Centroid", "Data PID"=w239) -> (w244:T6)
            n81 = Enqueue Element(queue=w246, element=w244, error in (no error)=w242) -> (error out=w241:errorcluster)  [unwired: 1 in, 2 out]
          }
          frame "Activer T-Cube" {
            w252 = T10 {"T-Cube X"=refnum, "T-Cube Y"=refnum}  # Référence T-Cube
            w256 = T6 {"Etat PID"=enum."PID", "Data PID"=variant}  # Data PID
            n82 = Unbundle By Name(w263) -> ("Data"=w261:variant)
            n83 = Variant To Data(error in=w262, type=FALSE, Variant=w261) -> (data=w259:bool, error out=w258:errorcluster)
            n84 = case shown="Vrai" w259 {
              tunnel: "TCube Axe X" -> [w271 w290]
              tunnel: [w269 w286] -> w264
              tunnel: w258 -> [w272 w289]
              tunnel: "SerialNumber Axe X" -> [_ w288]
              tunnel: w256 -> [_ w287]
              tunnel: w255 -> [_ w284]
              tunnel: "TCube Axe Y" -> [w268 w281]
              tunnel: "SerialNumber Axe Y" -> [_ w280]
              tunnel: w252 -> [_ w279]
              tunnel: [w267 w275] -> w251
              tunnel: w250 -> [w267 w276]
              frame False {
                n85 = invoke class="TCubePiezoControl" method="CloseDevice"(reference=w271, error in=w272) -> (error out=w270:errorcluster)  [unwired: 1 in, 2 out]
                n86 = invoke class="TCubePiezoControl" method="CloseDevice"(reference=w268, error in=w270) -> (error out=w269:errorcluster)  [unwired: 1 in, 2 out]
              }
              frame True {
                n87 = call "Init T-Cube.vi"("entrée d'erreur (pas d'erreur)"=w289, "SerialNumber"=w288, "Refnum de .NET en entrée"=w290) -> ("sortie d'erreur"=w282:errorcluster, "Refnum de .NET en sortie"=w274:refnum<k24>)  [unwired: 7 in]
                "Refnum de .NET en sortie" <- w274
                n88 = call "Init T-Cube.vi"("entrée d'erreur (pas d'erreur)"=w282, "SerialNumber"=w280, "Refnum de .NET en entrée"=w281) -> ("sortie d'erreur"=w277:errorcluster, "Refnum de .NET en sortie"=w273:refnum<k24>)  [unwired: 7 in]
                n89 = Bundle By Name(cluster=w276, "Référence T-Cube.T-Cube X"=w274, "Référence T-Cube.T-Cube Y"=w273) -> (w275:T8)
                n90 = Bundle By Name(cluster=w279, "T-Cube X"=w274, "T-Cube Y"=w273) -> (w278:T10)
                n91 = Bundle By Name(cluster=w287, "Etat PID"=Etat_PID."Set T-Cube", "Data PID"=w278) -> (w285:T6)
                n92 = Enqueue Element(queue=w284, element=w285, error in (no error)=w277) -> (error out=w286:errorcluster)  [unwired: 1 in, 2 out]
              }
            }
          }
        }
        n93 = Or(x=w64, y=w72) -> (x .or. y?=w73:bool)
      }
    }
    frame Error {
    }
  }
  n94 = while {
    tunnel: [w300] -> w43
    tunnel: w37 -> [w299]
    tunnel: [w298] -> w36
    tunnel: w35 -> [w297]
    tunnel: [w295] -> w11
    tunnel: w10 -> [w294]
    stop <- w296 stop-if-true
    # "Gestion de l'interface"
    n95 = event shown="[6] \"Shutter (us)\": Valeur changée" {
      selector: _ -> [_ _ _ _ _ _ _ _ _]
      dyn-events: _ -> [_ _ _ _ _ _ _ _ _]
      timeout: -1 -> [_ _ _ _ _ _ _ _ _]
      tunnel: [w303 w305 w320 w337 w349 w371 w379 w387 w409] -> w300
      tunnel: w299 -> [w303 w313 w321 w338 w348 w372 w380 w388 w410]
      tunnel: [w302 w307 w322 w335 w350 w370 w378 w386 w404] -> w298
      tunnel: w297 -> [w302 w312 w323 w336 w351 w369 w377 w385 w405]
      tunnel: [_ w308 _ _ _ _ _ _ _] -> w296
      tunnel: [_ _ w317 _ _ _ _ _ w403] -> w295
      tunnel: w294 -> [_ _ w317 _ _ _ _ _ w402]
      event Timeout {
        n96 = event-data() -> ()  [unwired: 1 in, 1 out]
      }
      event "stop": Value Change {
        w310 = T12 {"Etat"=enum."Initialiser", "Data"=variant}  # Etat/Data
        n97 = event-data() -> ()  [unwired: 1 in, 1 out]
        n98 = Bundle By Name(cluster=w310, "Etat"=Etat."Stop Prog") -> (w309:T12)
        n99 = Enqueue Element(queue=w313, element=w309, error in (no error)=w312) -> (queue out=w304:refnum<queue>, error out=w306:errorcluster)  [unwired: 1 in, 1 out]
        n100 = flat-sequence {
          tunnel: [TRUE] -> w308
          tunnel: [w315] -> w307
          tunnel: w306 -> [w315]
          tunnel: [w314] -> w305
          tunnel: w304 -> [w314]
          frame #0 {
          }
        }
      }
      event "Set Centroid": Value Change {
        n101 = event-data() -> ("NewVal"=w319:bool)  [unwired: 1 in, 2 out]
        n102 = case shown="Vrai" w319 {
          tunnel: w323 -> [w325 w331]
          tunnel: [w325 w330] -> w322
          tunnel: w321 -> [w326 w329]
          tunnel: [w326 w328] -> w320
          tunnel: [FALSE ("Set Centroid") FALSE ("Set Centroid")] -> w318
          frame False {
          }
          frame True {
            w333 = T12 {"Etat"=enum."Initialiser", "Data"=variant}  # Etat/Data
            n103 = Bundle By Name(cluster=w333, "Etat"=Etat."Set Centroid") -> (w334:T12)
            n104 = Enqueue Element(queue=w329, element=w334, error in (no error)=w331) -> (queue out=w328:refnum<queue>, error out=w330:errorcluster)  [unwired: 1 in, 1 out]
          }
        }
        n105 = local write "Set Centroid"(w318) -> ()
      }
      event "Start /Stop Acquisition": Value Change {
        w344 = T12 {"Etat"=enum."Initialiser", "Data"=variant}  # Etat/Data
        n106 = event-data() -> ("NewVal"=w343:bool)  [unwired: 1 in]
        n107 = Select(t=Etat."Start Acquisition" ("Etat"), s=w343, f=Etat."Stop Acquisition" ("Etat")) -> (s? t:f=w340:T11)
        n108 = Bundle By Name(cluster=w344, "Etat"=w340) -> (w339:T12)
        n109 = Enqueue Element(queue=w338, element=w339, error in (no error)=w336) -> (queue out=w337:refnum<queue>, error out=w335:errorcluster)  [unwired: 1 in, 1 out]
      }
      event "Bruit de fond": Value Change {
        n110 = event-data() -> ("NewVal"=w347:bool)  [unwired: 1 in]
        n111 = case shown="Vrai" w347 {
          tunnel: w351 -> [w356 w362]
          tunnel: [w356 w361] -> w350
          tunnel: [w357 w360] -> w349
          tunnel: w348 -> [w357 w359]
          tunnel: [FALSE ("Bruit de fond") FALSE ("Bruit de fond")] -> w345
          frame False {
          }
          frame True {
            w364 = T12 {"Etat"=enum."Initialiser", "Data"=variant}  # Etat/Data
            n112 = Bundle By Name(cluster=w364, "Etat"=Etat."BKG") -> (w365:T12)
            n113 = Enqueue Element(queue=w359, element=w365, error in (no error)=w362) -> (queue out=w360:refnum<queue>, error out=w361:errorcluster)  [unwired: 1 in, 1 out]
          }
        }
        n114 = flat-sequence {
          tunnel: [w353] -> w346
          tunnel: w345 -> [w354]
          frame #0 {
            n115 = call "Stall Data Flow.vim"("value in"=w354, "milliseconds to wait"=u32 200) -> ("value out"=w353:bool)  [unwired: 1 out]
          }
        }
        n116 = local write "Bruit de fond"(w346) -> ()
      }
      event "Gain Caméra": Value Change {
        w368 = T12 {"Etat"=enum."Initialiser", "Data"=variant}  # Etat/Data
        n117 = event-data() -> ("NewVal"=w366:i32)  [unwired: 1 in]
        n118 = Bundle By Name(cluster=w368, "Etat"=Etat."Gain", "Data"=w366) -> (w367:T12)
        n119 = Enqueue Element(queue=w372, element=w367, error in (no error)=w369) -> (queue out=w371:refnum<queue>, error out=w370:errorcluster)  [unwired: 1 in, 1 out]
      }
      event "Shutter (us)": Value Change {
        w376 = T12 {"Etat"=enum."Initialiser", "Data"=variant}  # Etat/Data
        n120 = event-data() -> ("NewVal"=w374:dbl)  [unwired: 1 in]
        n121 = Bundle By Name(cluster=w376, "Etat"=Etat."Shutter", "Data"=w374) -> (w375:T12)
        n122 = Enqueue Element(queue=w380, element=w375, error in (no error)=w377) -> (queue out=w379:refnum<queue>, error out=w378:errorcluster)  [unwired: 1 in, 1 out]
      }
      event "Save Image": Value Change {
        n123 = event-data() -> ("NewVal"=w384:bool)  [unwired: 1 in]
        n124 = case shown="Vrai" w384 {
          tunnel: w388 -> [w392 w400]
          tunnel: [w392 w399] -> w387
          tunnel: [w391 w398] -> w386
          tunnel: w385 -> [w391 w397]
          tunnel: [FALSE ("Save Image") FALSE ("Save Image")] -> w383
          frame False {
          }
          frame True {
            w396 = T12 {"Etat"=enum."Initialiser", "Data"=variant}  # Etat/Data
            n125 = Bundle By Name(cluster=w396, "Etat"=Etat."Save Image") -> (w395:T12)
            n126 = Enqueue Element(queue=w400, element=w395, error in (no error)=w397) -> (queue out=w399:refnum<queue>, error out=w398:errorcluster)  [unwired: 1 in, 1 out]
          }
        }
        n127 = flat-sequence {
          tunnel: w383 -> [w389]
          tunnel: [w389] -> w382
          frame #0 {
            n128 = Wait Until Next ms Multiple(millisecond multiple=u32 1000 ("n millisecondes")) -> ()  [unwired: 1 out]
          }
        }
        n129 = local write "Save Image"(w382) -> ()
      }
      event "Activer T-CUbe": Value Change {
        w407 = T12 {"Etat"=enum."Initialiser", "Data"=variant}  # Etat/Data
        n130 = event-data() -> ("NewVal"=w408:bool)  [unwired: 1 in]
        n131 = case shown="Faux" w408 {
          selector: w408 -> [w414 w426]
          tunnel: w410 -> [w419 w428]
          tunnel: [w418 w427] -> w409
          tunnel: w407 -> [w413 w425]
          tunnel: Etat."Activer T-Cube" ("Etat") -> [w415 w423]
          tunnel: w405 -> [w417 w422]
          tunnel: [w416 w421] -> w404
          tunnel: [w411 w420] -> w403
          tunnel: w402 -> [w411 w420]
          frame False {
            n132 = Bundle By Name(cluster=w413, "Etat"=w415, "Data"=w414) -> (w412:T12)
            n133 = Enqueue Element(queue=w419, element=w412, error in (no error)=w417) -> (queue out=w418:refnum<queue>, error out=w416:errorcluster)  [unwired: 1 in, 1 out]
          }
          frame True {
            n134 = Bundle By Name(cluster=w425, "Etat"=w423, "Data"=w426) -> (w424:T12)
            n135 = Enqueue Element(queue=w428, element=w424, error in (no error)=w422) -> (queue out=w427:refnum<queue>, error out=w421:errorcluster)  [unwired: 1 in, 1 out]
          }
        }
      }
    }
  }
  n136 = while {
    tunnel: w10 -> [w442]
    shift-right: [w438] -> _
    shift-left: FALSE -> [w437]
    tunnel: [w435] -> _
    shift-right: [w434] -> _
    shift-left: w8 -> [w433]
    shift-right: [w432] -> _
    shift-left: w6 -> [w431]
    shift-right: [w430] -> _
    shift-left: w6 -> [w429]
    stop <- w439 stop-if-true
    # "Processus PID"
    n137 = Dequeue Element(queue=w442) -> (element=w441:T6, error out=w436:errorcluster)  [unwired: 2 in, 2 out]
    n138 = Unbundle By Name(w441) -> ("Etat PID"=w440:T7)
    n139 = case shown="\"Set Centroid\"" w440 {
      tunnel: w441 -> [w468 _ w496 w505 _]
      tunnel: [_ _ _ _ TRUE] -> w439
      tunnel: [w466 TRUE w497 w507 w512] -> w438
      tunnel: w437 -> [w466 _ w497 w507 w512]
      tunnel: w436 -> [w465 w483 w494 w503 w511]
      tunnel: [w460 w483 w493 w502 w511] -> w435
      tunnel: [w464 w482 w491 w506 w510] -> w434
      tunnel: w433 -> [w464 w482 w492 w506 w510]
      tunnel: [w446 w481 w490 w499 w509] -> w432
      tunnel: w431 -> [w447 w481 w490 _ w509]
      tunnel: [w449 w480 w489 w498 w508] -> w430
      tunnel: w429 -> [w461 w480 w489 _ w508]
      frame "PID", Default {
        n140 = Unbundle By Name(w468) -> ("Data PID"=w467:variant)
        n141 = Variant To Data(error in=w465, type=cluster{dbl, dbl} {0.0, 0.0} ("cluster"), Variant=w467) -> (data=w455:cluster{dbl, dbl}, error out=w444:errorcluster)
        n142 = Unbundle By Name(w464) -> ("Pos Init CX"=w463:dbl, "Pos Init CY"=w450:dbl)
        n143 = Unbundle(w455) -> (w454:dbl, w451:dbl)
        n144 = Subtract(x=w454, y=w463) -> (x-y=→"CX-offset":dbl)
        n145 = Subtract(x=w451, y=w450) -> (x-y=w448:dbl)
        "CY-offset" <- w448
        n146 = disable-structure shown="Activé" {
          disable-tunnel: w447 -> [w477 w479]
          disable-tunnel: [w476 w479] -> w446
          disable-tunnel: [w475 w478] -> w445
          disable-tunnel: w444 -> [w474 w478]
          disable-tunnel: _ -> [w473 _]
          disable-tunnel: _ -> [w472 _]
          disable-tunnel: _ -> [w471 _]
          disable-tunnel: _ -> [w470 _]
          disable-tunnel: _ -> [w469 _]
          frame Disabled {
            n147 = call "Start PID.vi"("Reset PID en entrée"=w471, "dt (s) PID"=w472, "Centroid Variable"=w470, "entrée d'erreur (pas d'erreur)"=w474, "PID gains"=w473, "Switch Axe"=w469, "Refnum de .NET en entrée"=w477) -> ("sortie d'erreur"=w475:errorcluster, "Refnum de .NET en sortie"=w476:refnum<k24>)  [unwired: 2 in, 1 out]
          }
          frame Enabled {
          }
        }
        n148 = call "Start PID.vi"("Reset PID en entrée"="Reset PID 2", "dt (s) PID"="dt (s) PID Axe Y", "Centroid Variable"=w448, "entrée d'erreur (pas d'erreur)"=w444, "PID gains"="PID gains Axe Y", "Switch Axe"="Switch Axe Y", "Refnum de .NET en entrée"=w461) -> ("sortie d'erreur"=w462:errorcluster, "Tension Sortie PID"=→"Tension Sortie PID Axe Y":dbl, "Refnum de .NET en sortie"=w449:refnum<k24>)  [unwired: 2 in]
        n149 = Merge Errors(w445, w462) -> (w460:errorcluster)
      }
      frame "Reset PID" {
      }
      frame "Set Centroid" {
        n150 = Unbundle By Name(w496) -> ("Data PID"=w495:variant)
        n151 = Variant To Data(error in=w494, type=T13 {"CX"=0.0, "CY"=0.0} ("cluster"), Variant=w495) -> (data=w487:T13, error out=w493:errorcluster)
        n152 = Unbundle By Name(w487) -> ("CX"=w486:dbl, "CY"=w485:dbl)
        "Set CX" <- w486
        "Set CY" <- w485
        n153 = Bundle By Name(cluster=w492, "Pos Init CX"=w486, "Pos Init CY"=w485) -> (w491:T5)
      }
      frame "Set T-Cube" {
        w501 = T10 {"T-Cube X"=refnum, "T-Cube Y"=refnum}  # Référence T-Cube
        n154 = Unbundle By Name(w505) -> ("Data PID"=w504:variant)
        n155 = Variant To Data(error in=w503, type=w501, Variant=w504) -> (data=w500:T10, error out=w502:errorcluster)
        n156 = Unbundle By Name(w500) -> ("T-Cube X"=w499:refnum<k24>, "T-Cube Y"=w498:refnum<k24>)
      }
      frame "Stop" {
      }
    }
  }
  n157 = Release Queue(queue=w43, error in (no error)=w36) -> (error out=w12:errorcluster)  [unwired: 1 in, 2 out]
  n158 = Release Queue(queue=w11, error in (no error)=w12) -> ()  [unwired: 1 in, 3 out]
  n159 = Unbundle By Name(w16) -> ("Camera"=w15:refnum<class "Camera.lvclass">, "Buffer en sortie"=w14:refnum<class "Buffer.lvclass">)
  n160 = call <vilib>:"Destroy.vi"("error in (no error)"=w45, "Buffer in"=w14) -> ("error out"=w44:errorcluster)  [unwired: 9 in]
  n161 = flat-sequence {
    tunnel: [w514] -> w33
    tunnel: w32 -> [w514]
    frame #0 {
      n162 = Wait (ms)(milliseconds to wait=u32 500 ("attente (ms)")) -> ()  [unwired: 1 out]
    }
  }
  n163 = call <vilib>:"Destroy.vi"("error in (no error)"=w44, "Camera in"=w15) -> ("error out"=→"error out":errorcluster)  [unwired: 9 in]
  n164 = Not(x=w33) -> (.not. x?=w34:bool)
  n165 = local write "stop"(w34) -> ()
